vi "CLI Help--constant.vi"() -> (3 "Help Message":string)   [LabVIEW 2025]
doc: "Help message for CLI."
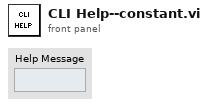
[diagram p1: front panel]
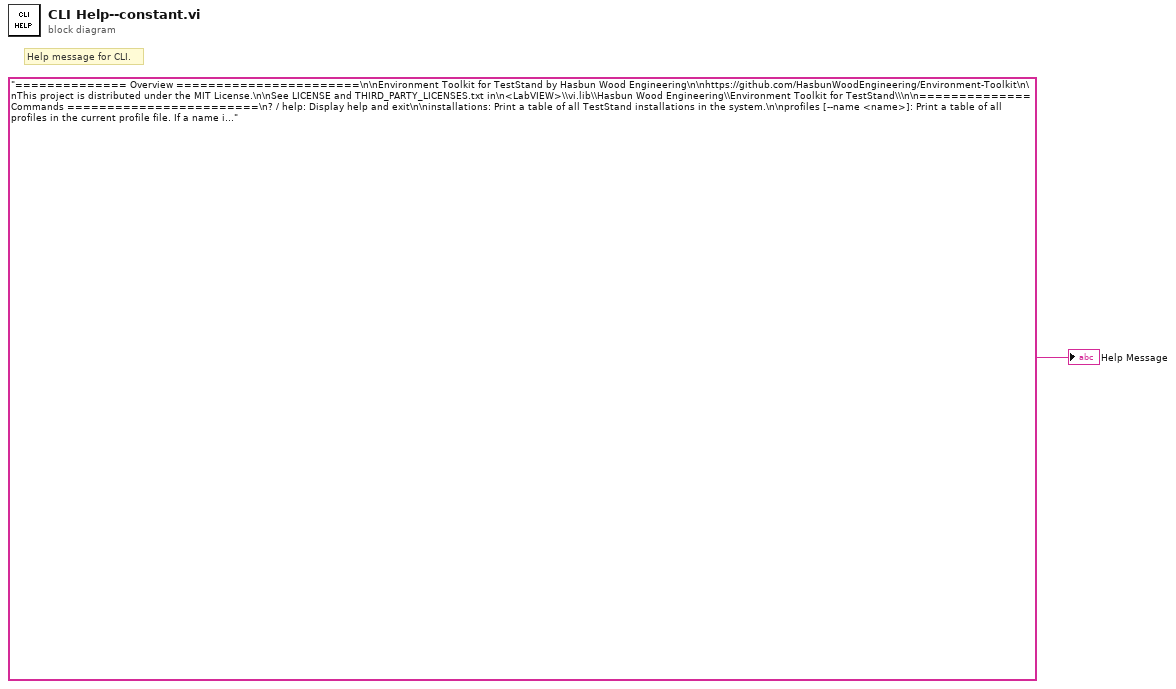
[diagram p0: block diagram]
diagram:
  # "Help message for CLI."
  "Help Message" <- "============== Overview =======================\n\nEnvironment Toolkit for TestStand by Hasbun Wood Engineering\n\nhttps://github.com/HasbunWoodEngineering/Environment-Toolkit\n\nThis project is distributed under the MIT License.\n\nSee LICENSE and THIRD_PARTY_LICENSES.txt in\n<LabVIEW>\\vi.lib\\Hasbun Wood Engineering\\Environment Toolkit for TestStand\\\n\n============== Commands ========================\n? / help: Display help and exit\n\ninstallations: Print a table of all TestStand installations in the system.\n\nprofiles [--name <name>]: Print a table of all profiles in the current profile file. If a name is provided only the specified profile will be printed.\n\nopen: Open the active profiles file in notepad.exe.\n\nnew --name <name> --version <version> --arch <architecture> [--file <environment>]: Create a new profile in the current file. Environment is an optional parameter.\n\ndelete --name <name>: Delete profile from current file.  \n\nset-file --file <profiles.ini>: Set profiles file.\n\nlaunch --name <name>: Launch the specified profile. This will activate the profiles TestStand version (if necessary) and launch the sequence editor with the corresponding environment.\n\nactivate --version <version>: Activate the specified TestStand version.\n\nlicenses: display license information of the project.\n\n=============== Examples =====================\n\nCreate a profile:\ng-cli --lv-ver 2025 --arch 32  --kill env-toolkit -- new --name customer1-project1 --version 25.5 --arch 64 --file C:\\Users\\Public\\Documents\\development.tsenv\n\nLaunch:\ng-cli --lv-ver 2025 --arch 32  --kill env-toolkit -- launch --name customer1-project1\n============================================"
